vi "Untitled 2.vi"(1 "Numeric":i32) -> (0 "Array":i32[](array[numeric]))   [LabVIEW 2015]
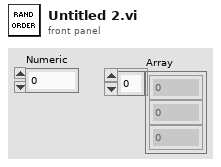
[diagram p1: front panel]
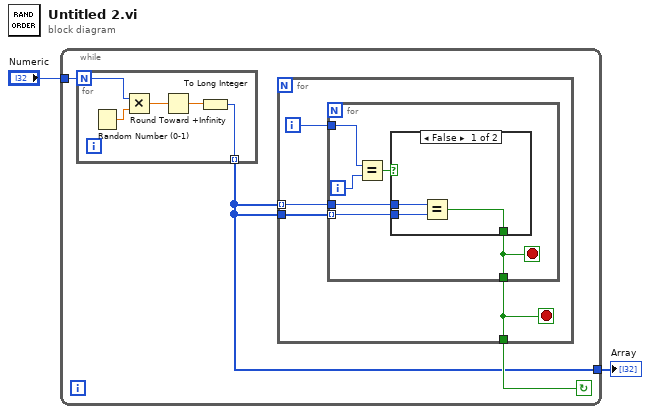
[diagram p0: block diagram]
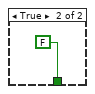
[diagram p2: hidden frame]
diagram:
  n1 = while {
    tunnel: "Numeric" -> [w5]
    tunnel: [w3] -> w1
    stop <- w4 continue-if-true
    n2 = for {
      N: w5 -> [w23]
      tunnel: [w20] -> w3 mode=indexing
      n3 = Random Number (0-1)() -> (number: 0 to 1=w24:dbl)
      n4 = Multiply(x=w23, y=w24) -> (x*y=w22:dbl)
      n5 = Round Toward +Infinity(x=w22) -> (ceil(x): smallest int >= x=w21:dbl)
      n6 = To Long Integer(number=w21) -> (32bit integer=w20:i32)
    }
    n7 = for {
      tunnel: [w8] -> w4
      tunnel: w3 -> [w7] mode=indexing
      tunnel: w3 -> [w6]
      i -> [w9]
      stop <- w8 stop-if-true
      n8 = for {
        tunnel: w9 -> [w14]
        tunnel: [w12] -> w8
        tunnel: w7 -> [w11]
        tunnel: w6 -> [w10] mode=indexing
        i -> [w15]
        stop <- w12 stop-if-true
        n9 = Equal?(x=w14, y=w15) -> (x = y?=w13:bool)
        n10 = case shown="False" w13 {
          tunnel: [w18 FALSE] -> w12
          tunnel: w11 -> [w17 _]
          tunnel: w10 -> [w16 _]
          frame False {
            n11 = Equal?(x=w17, y=w16) -> (x = y?=w18:bool)
          }
          frame True {
          }
        }
      }
    }
  }
  "Array" <- w1
